vi "getposition.vi"(8 "error in (no error)":errorcluster, 11 "VISA resource name":refnum<visa-resource-name>) -> (0 "error out":errorcluster, 1 "Is Null?":bool, 2 "Position":i32, 3 "VISA resource name 2":refnum<visa-resource-name>)   [LabVIEW 2019]
panel:
  out "bytes":u32
  out "return count":u32
  out "read buffer":string
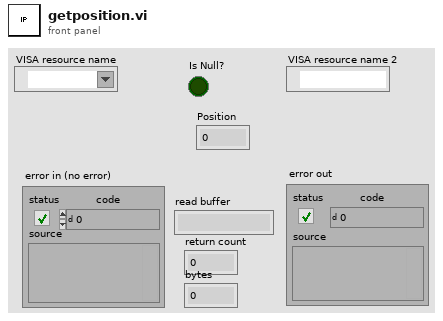
[diagram p1: front panel]
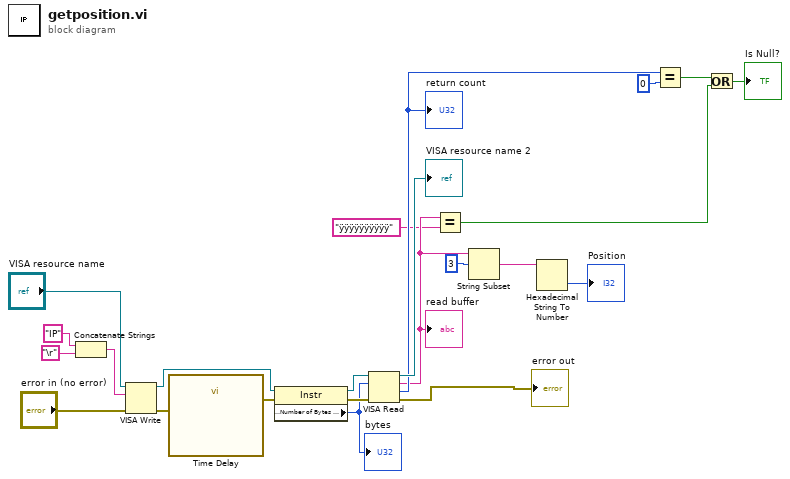
[diagram p0: block diagram]
diagram:
  n1 = Concatenate Strings("IP", "\r") -> (w21:string)
  n2 = VISA Write(VISA resource name="VISA resource name", write buffer=w21, error in (no error)="error in (no error)") -> (VISA resource name out=w7:refnum<visa-resource-name>, error out=w3:errorcluster)  [unwired: 1 out]
  n3 = call "Time Delay"("error in (no error)"=w3) -> ("error out"=w2:errorcluster)  [unwired: 10 in]
  n4 = property class="Instr"(reference=w7, error in=w2) -> (reference out=w6:refnum<visa-resource-name>, error out=w5:errorcluster, "Serial Settings:Number of Bytes at Serial Port"=w4:u32)
  "bytes" <- w4
  n5 = VISA Read(VISA resource name=w6, byte count=w4, error in (no error)=w5) -> (VISA resource name out=→"VISA resource name 2":refnum<visa-resource-name>, read buffer=w12:string, return count=w14:u32, error out=→"error out":errorcluster)
  "read buffer" <- w12
  "return count" <- w14
  n6 = Equal?(x=w12, y="ÿÿÿÿÿÿÿÿÿÿ") -> (x = y?=w9:bool)
  n7 = String Subset(string=w12, offset (0)=3) -> (substring=w17:string)  [unwired: 1 in]
  n8 = Hexadecimal String To Number(string=w17) -> (number=→"Position":u32)  [unwired: 2 in, 1 out]
  n9 = Equal?(x=w14, y=u32 0) -> (x = y?=w10:bool)
  n10 = Or(x=w10, y=w9) -> (x .or. y?=→"Is Null?":bool)
